vi "Load Last Scan.vi"(8 "error in":errorcluster) -> (0 "error out":errorcluster, 3 "Last Run Scan":refnum<class "Scan Driver.lvclass">)   [LabVIEW 2009, in "File IO.lvclass"]
doc: "Attempts to load the scan from the \"Last Run\" file. If the scan is missing, prompts the user to find it. If an error occurs while loading a file, the class default object is returned."
uses:
  File IO.lvclass
  Main/Scan Driver/Scan Driver.lvclass
  Global/File Locations.vi
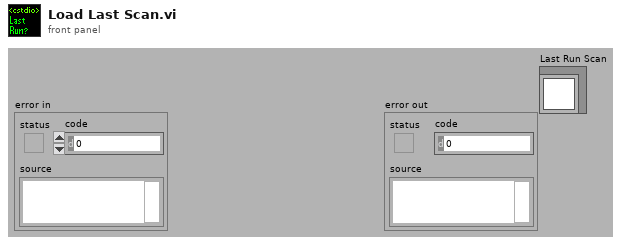
[diagram p1: front panel]
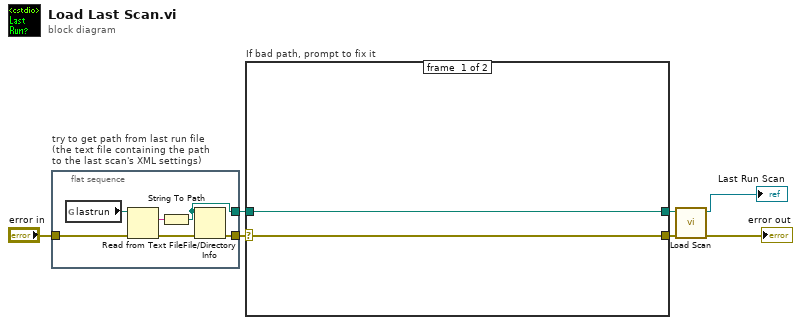
[diagram p0: block diagram]
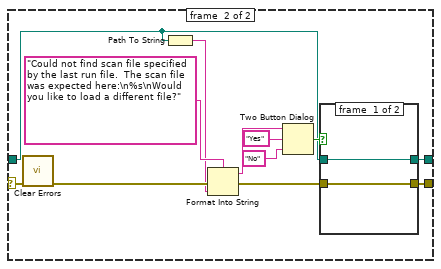
[diagram p2: hidden frame]
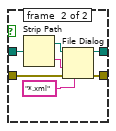
[diagram p3: hidden frame]
diagram:
  n1 = flat-sequence "try to get path from last run file\n(the text file containing the path\nto the last scan's XML settings)" {
    tunnel: [w13] -> w7
    tunnel: "error in" -> [w10]
    tunnel: [w8] -> w5
    frame #0 {
      n2 = global read "File Locations.vi" "lastrun"() -> (w11:path)
      n3 = Read from Text File(file (use dialog)=w11, error in=w10) -> (text=w12:string, error out=w9:errorcluster)  [unwired: 4 out]
      n4 = String To Path(string=w12) -> (path=w13:path)
      n5 = File/Directory Info(path=w13, error in=w9) -> (error out=w8:errorcluster)  [unwired: 6 out]
    }
  }
  n6 = case "If bad path, prompt to fix it" shown="Error" w5 {
    selector: w5 -> [w14 w21]
    tunnel: w7 -> [w15 w23]
    tunnel: [w15 w24] -> w3
    tunnel: [w14 w22] -> w4
    frame #0 {
    }
    frame #1 {
      n7 = call <vilib>:"Clear Errors.vi"("error in (no error)"=w21) -> ("error out"=w19:errorcluster)  [unwired: 6 out]
      n8 = Path To String(path=w23) -> (string=w17:string)
      n9 = Format Into String(format string="Could not find scan file specified by the last run file.  The scan file was expected here:\n%s\nWould you like to load a different file?", error in=w19, w17) -> (resulting string=w16:string, error out=w18:errorcluster)  [unwired: 1 in]
      n10 = Two Button Dialog(message=w16, 1:"No", 2:"Yes") -> (T button?=w25:bool)
      n11 = case shown="True" w25 {
        tunnel: [w29 w36] -> w24
        tunnel: w23 -> [w29 w33]
        tunnel: w18 -> [w28 w32]
        tunnel: [w28 w31] -> w22
        frame #0 {
        }
        frame #1 {
          n12 = Strip Path(path=w33) -> (stripped path=w35:path, name=w34:string)
          n13 = File Dialog(6:"*.xml" ("pattern (all files)"), 8:w32, 9:w34, 11:w35) -> (0:w31:errorcluster, 3:w36:path)  [unwired: 5 out]
        }
      }
    }
  }
  n14 = call "Load Scan.vi"("error in (no error)"=w4, "XML File Path"=w3) -> ("error out"=→"error out":errorcluster, "Scan Driver out"=→"Last Run Scan":refnum<class "Scan Driver.lvclass">)  [unwired: 8 out]
